vi "turning_correction.vi"(9 "Parâmetros Ini 2":T1={"Gyro Port"=0, "Sensor - Left"=3, "Sensor - Right"=2, "     Color \nSensor Port"=1, "Kp Front"=0.5, "Motor speed"=-15, "Distance to street"=0.0, "Motor speed turns"=16, "Kp Curvas"=0.0} {"Kp Front" format="%.3f"; "Color \nSensor Port" items=["Port 1", "Port 2", "Port 3", "Port 4"]; "Sensor - Right" items=["Port 1", "Port 2", "Port 3", "Port 4"]; "Sensor - Left" items=["Port 1", "Port 2", "Port 3", "Port 4"]; "Gyro Port" items=["Port 1", "Port 2", "Port 3", "Port 4"]}, 11 "NXT/EV3":T3) -> (1 "NXT/EV3 2":T3)   [LabVIEW 2016]
uses:
  <vilib>/NXT/Subs/LVHSConnector.ctl
  <vilib>/NXT/LegoClasses/BrickReference/BrickReference.lvclass
  parametros.ctl
  <vilib>/NXT/Block Support/NXT_InputPort.ctl
  <vilib>/NXT/Block Support/NXT_OutputPort.ctl
  <vilib>/NXT/Subs/ColorSensorColors.ctl
  <vilib>/NXT/Dual Mode Library/Display/drawText.vi
  <vilib>/NXT/Dual Mode Library/Sensors/EV3_Gyro_Angle.vi
  <vilib>/NXT/NXTIO Xnodes/NXTIONodeSubVIs/NXTMoveMotors.vi
  <vilib>/NXT/NXTIO Xnodes/NXTIONodeSubVIs/NXTMotorRunDistance.vi
  <vilib>/NXT/NXTIO Xnodes/AddressXNode/NXTIOAddress.xnode
  <vilib>/NXT/NXTIO Xnodes/NXTIOXNode/NXTIO.xnode
panel:
  out "Degrees":sgl
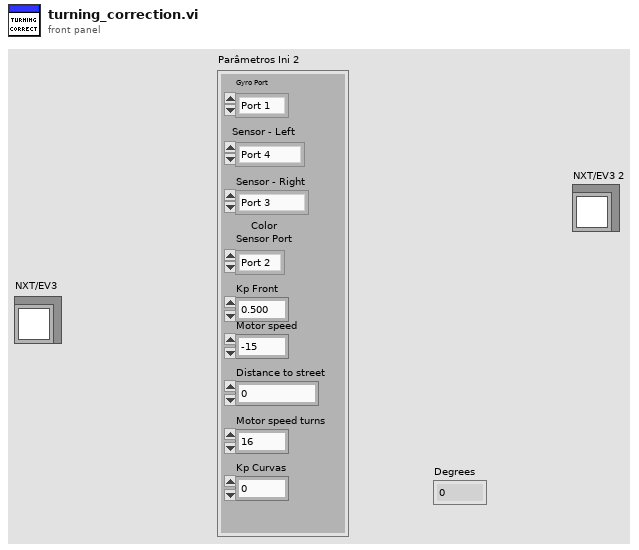
[diagram p1: front panel]
types:
  T1 = typedef "parametros.ctl" = cluster{"Gyro Port":T2, "Sensor - Left":T2, "Sensor - Right":T2, "     Color \nSensor Port":T2, "Kp Front":dbl, "Motor speed":i32, "Distance to street":dbl, "Motor speed turns":i32, "Kp Curvas":dbl}
  T2 = typedef "NXT_InputPort.ctl" = u32
  T3 = typedef "LVHSConnector.ctl" = refnum<class "BrickReference.lvclass">
  T4 = typedef "NXT_OutputPort.ctl" = u8
  T5 = typedef "ColorSensorColors.ctl" = enum16{"No Color", "Black", "Blue", "Green", "Yellow", "Red", "White", "Brown"}
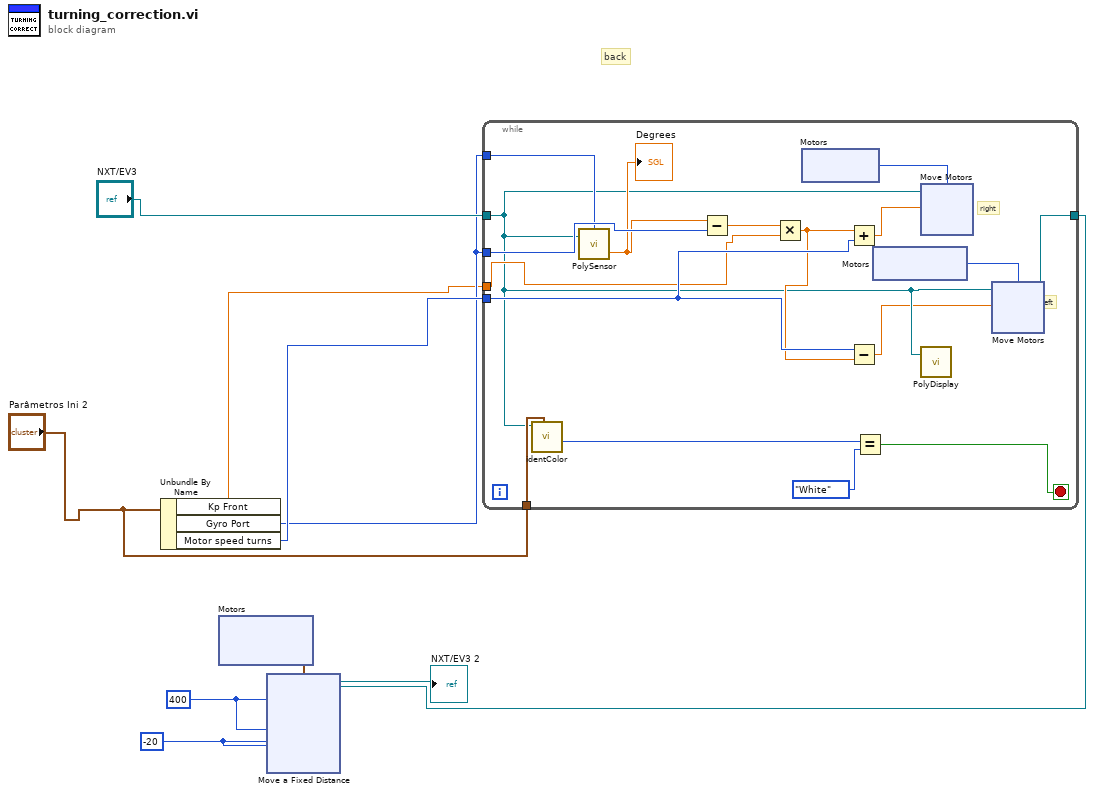
[diagram p0: block diagram]
diagram:
  w7 = i8 -20 ("Speed 1")
  w8 = 400 ("Distance 1")
  # "back"
  n1 = Unbundle By Name("Parâmetros Ini 2") -> ("Kp Front"=w3:dbl, "Gyro Port"=w4:T2, "Motor speed turns"=w5:i32)
  n2 = xnode "Motors"() -> ("Motor"=w9:cluster{"Port":T4, "Port":T4})
  n3 = while {
    tunnel: w4 -> [w27]
    tunnel: w5 -> [w26]
    tunnel: w4 -> [w25]
    tunnel: w3 -> [w24]
    tunnel: "Parâmetros Ini 2" -> [w15]
    tunnel: "NXT/EV3" -> [w13]
    tunnel: [w23] -> w2
    stop <- w16 stop-if-true
    # "left"
    # "right"
    n4 = call "identColor.vi"("Parâmetros Ini"=w15, "NXT/EV3"=w13) -> ("Collor"=w14:T5)  [unwired: 9 in]
    n5 = call-poly <vilib>:"PolySensor.vi"("NXT/EV3"=w13, "Port (Port 1)"=w25) -> ("Degrees"=w20:sgl)  [unwired: 1 in, 1 out]
    "Degrees" <- w20
    n6 = Subtract(x=w20, y=w27) -> (x-y=w21:sgl)
    n7 = Multiply(x=w21, y=w24) -> (x*y=w22:dbl)
    n8 = xnode "Motors"() -> ("Motor"=w19:T4)
    n9 = Add(x=w22, y=w26) -> (x+y=w12:dbl)
    n10 = Subtract(x=w26, y=w22) -> (x-y=w11:dbl)
    n11 = Equal?(x=w14, y=ColorSensorColors."White" ("Collor")) -> (x = y?=w16:bool)
    n12 = xnode "Motors"() -> ("Motor"=w18:T4)
    n13 = xnode "Move Motors"("Power/Speed 1"=w12, "Motors"=w19, "NXT/EV3"=w13) -> ()  [unwired: 1 out]
    n14 = call-poly <vilib>:"PolyDisplay.vi"("NXT/EV3"=w13) -> ()  [unwired: 3 in, 1 out]
    n15 = xnode "Move Motors"("Power/Speed 1"=w11, "Motors"=w18, "NXT/EV3"=w13) -> ("NXT/EV3"=w23:T3)
  }
  n16 = xnode "Move a Fixed Distance"("Speed 2"=w7, "Speed 1"=w7, "Distance 2"=w8, "Distance 1"=w8, "Motors"=w9, "NXT/EV3"=w2) -> ("NXT/EV3"=→"NXT/EV3 2":T3)
